vi "plot_data_update.vi"(0 "plotData":i32[][](array[numeric]), 1 "idx start":i32, 2 "length":i32, 3 "AcqData":sgl[](array[numeric]) format="%.2f", 5 "error in (no error)":errorcluster, 6 "max value":sgl format="%.2f", 7 "error rangeViolation":bool=TRUE, 8 "min value":sgl format="%.2f", 9 "error if all equal (false)":bool, 10 "autoScale Y":bool) -> (11 "pixels Y":i32, 13 "pixels X":i32, 14 "plotData out":i32[][](array[numeric]), 15 "updated":bool, 16 "length copy":u32, 17 "dataVal max":sgl format="%.2f", 18 "dataVal min":sgl format="%.2f", 19 "error out":errorcluster)   [LabVIEW 2010, in "OSA.lvclass"]
doc: "Reads the contents of a <B>Thorlabs_OSA_32</B> object.\n\n[GOOP 1.0]"
uses:
  OSA.lvclass
  OSA20X_misc.lvlib
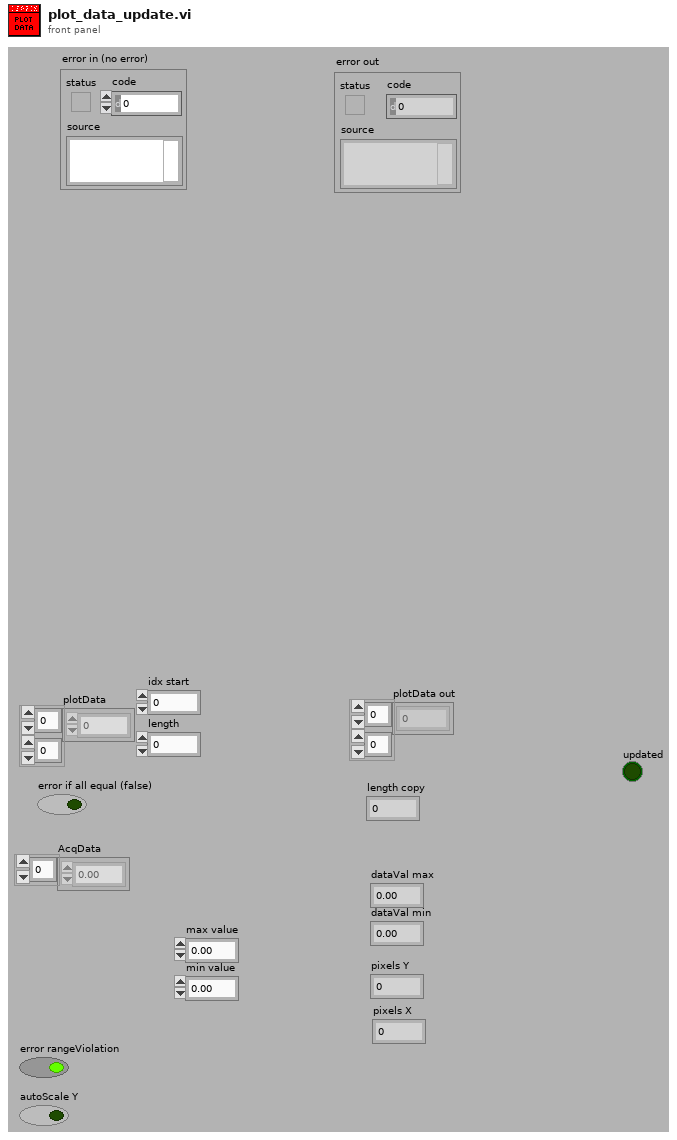
[diagram p1: front panel]
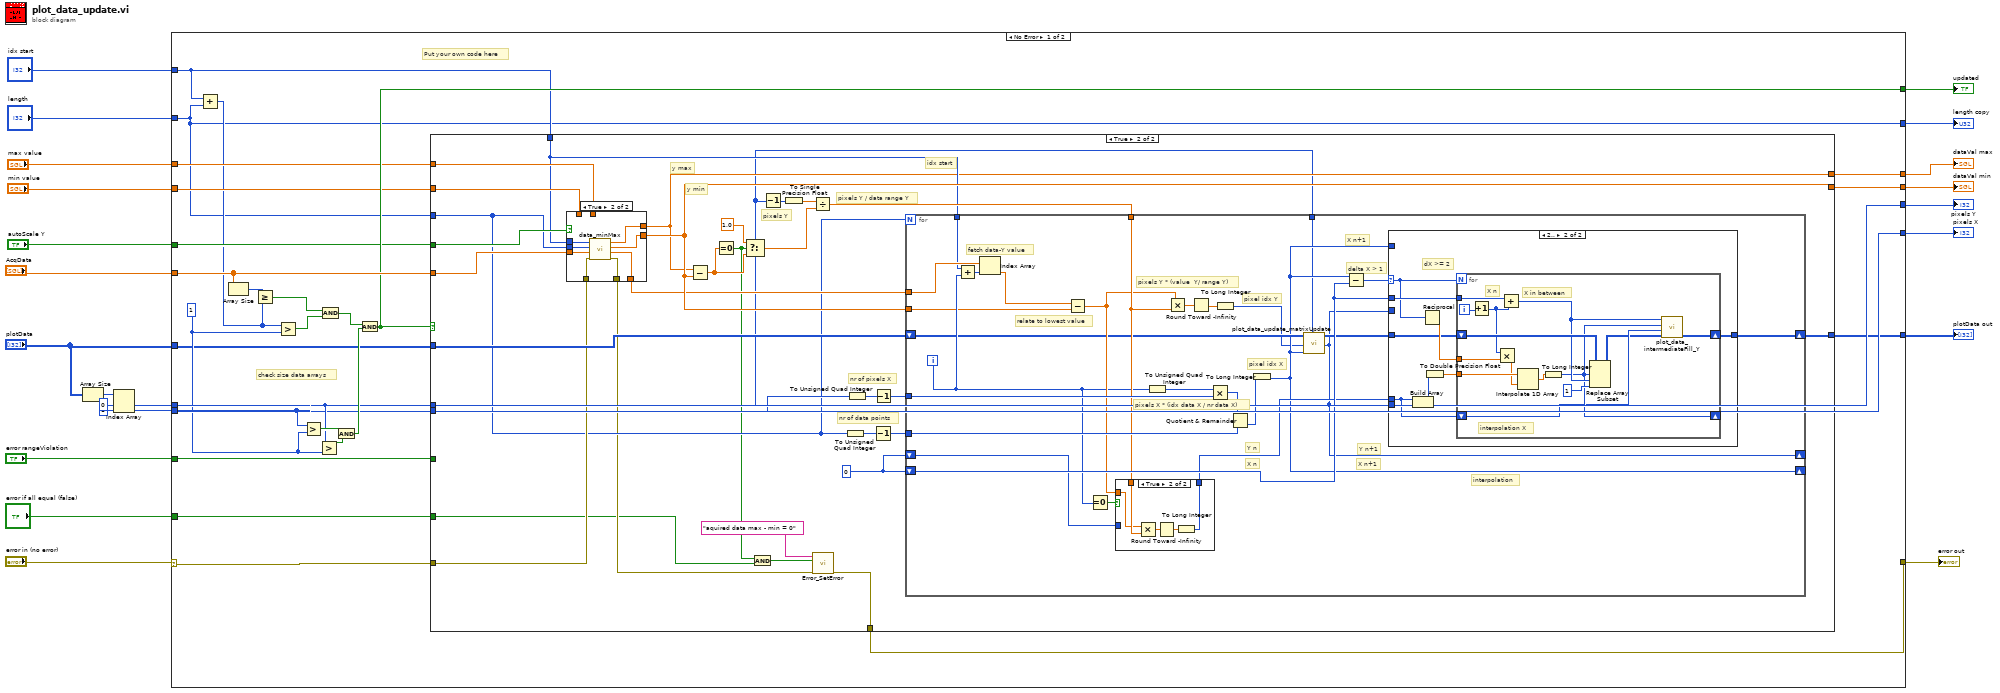
[diagram p0: block diagram]
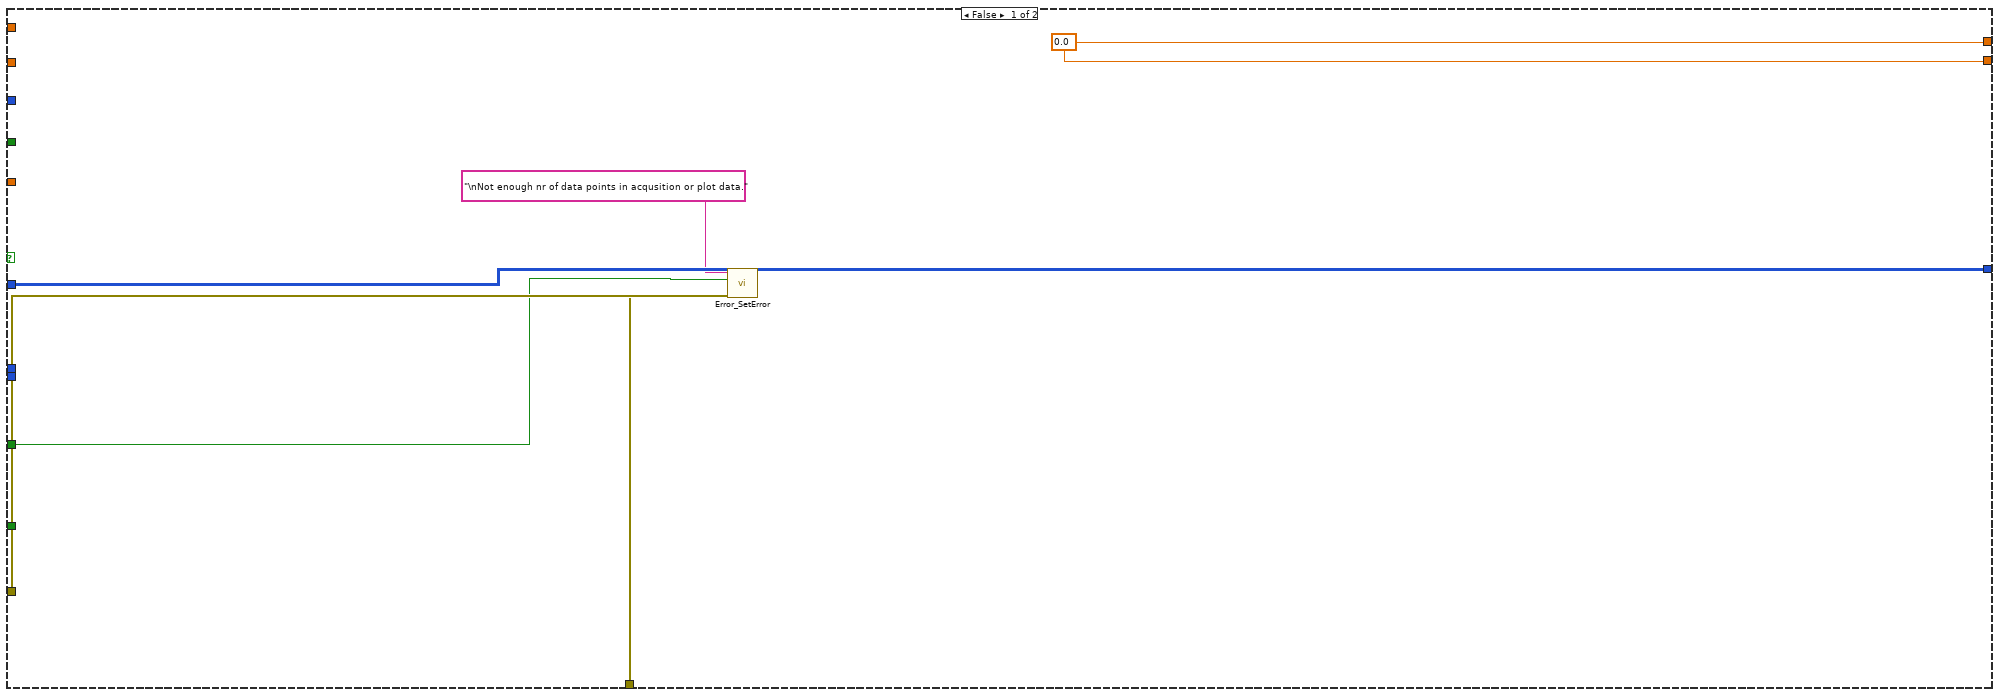
[diagram p2: hidden frame]
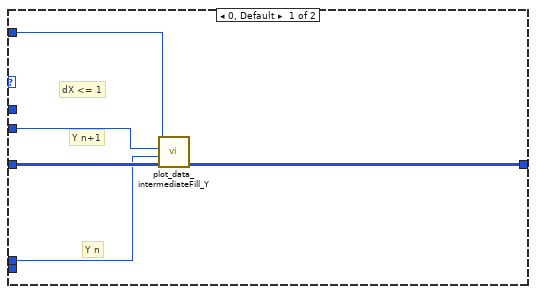
[diagram p5: hidden frame]
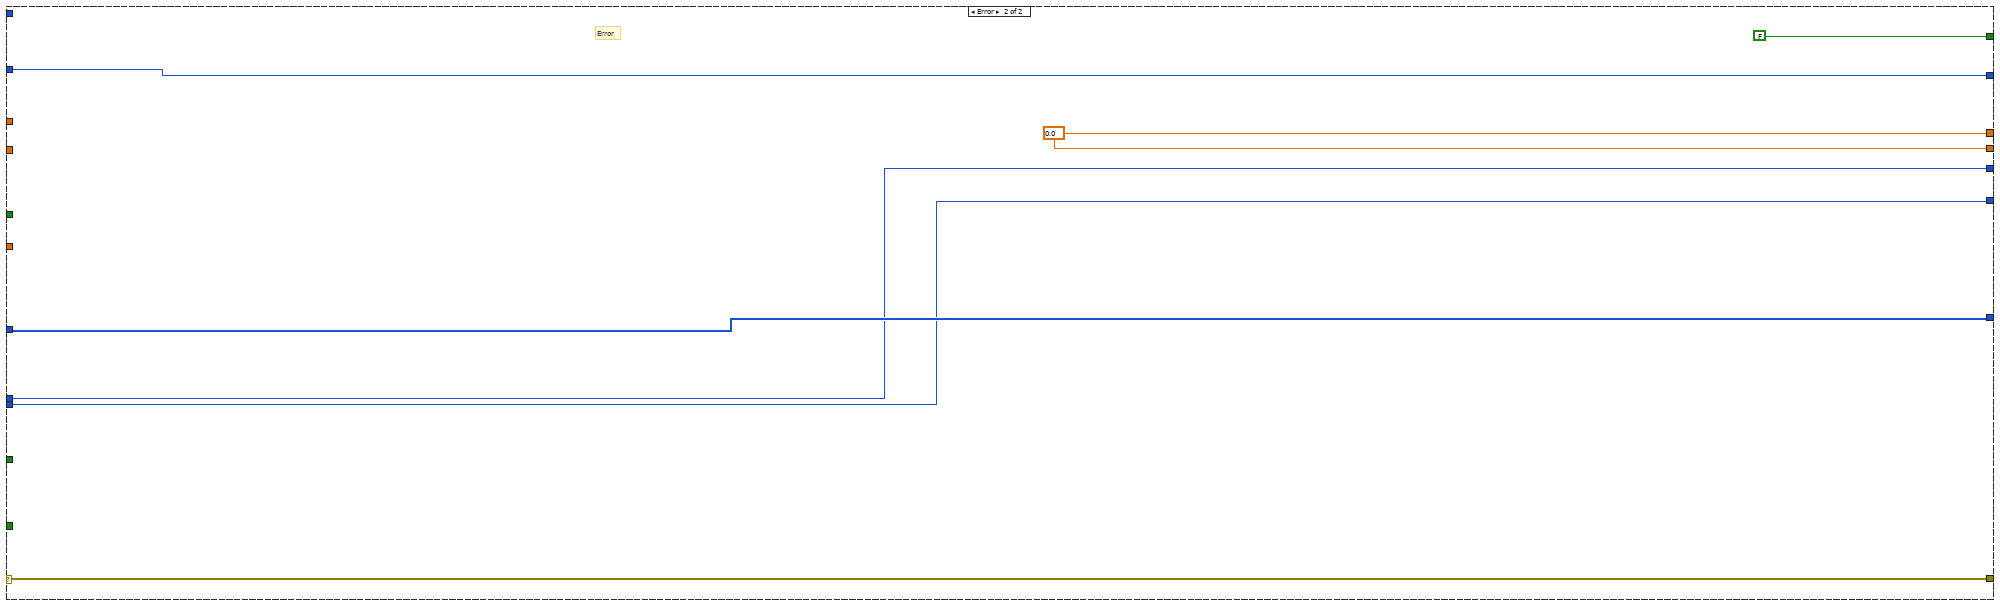
[diagram p6: hidden frame]
diagram:
  n1 = Array Size(array="plotData") -> (size(s)=w15:i32[])
  n2 = Index Array(array=w15, index #1=0 ("index"), index #2=1 ("index")) -> (element #1=w12:i32, element #2=w11:i32)
  n3 = case shown="No Error" "error in (no error)" {
    selector: "error in (no error)" -> [w40 w166]
    tunnel: [w39 w166] -> w23
    tunnel: "AcqData" -> [w49 _]
    tunnel: "plotData" -> [w34 w165]
    tunnel: [w33 w165] -> w2
    tunnel: [w38 w164] -> w20
    tunnel: [w37 w164] -> w19
    tunnel: [w25 w160] -> w18
    tunnel: [w36 w163] -> w17
    tunnel: [w35 w162] -> w16
    tunnel: w12 -> [w36 w163]
    tunnel: w11 -> [w35 w162]
    tunnel: "error rangeViolation" -> [w32 _]
    tunnel: [w31 FALSE] -> w8
    tunnel: "min value" -> [w30 _]
    tunnel: "max value" -> [w29 _]
    tunnel: "autoScale Y" -> [w28 _]
    tunnel: "idx start" -> [w27 _]
    tunnel: "length" -> [w25 w160]
    tunnel: "error if all equal (false)" -> [w24 _]
    frame No Error {
      w45 = u32 1 ("y")
      # "check size data arrays"
      # "Put your own code here"
      n4 = Add(x=w27, y=w25) -> (x+y=w26:i32)
      n5 = Array Size(array=w49) -> (size(s)=w48:i32)
      n6 = Greater Or Equal?(x=w48, y=w26) -> (x >= y?=w47:bool)
      n7 = Greater?(x=w26, y=w45) -> (0:w46:bool)
      n8 = Greater?(x=w35, y=w45) -> (0:w43:bool)
      n9 = Greater?(x=w36, y=w45) -> (0:w44:bool)
      n10 = And(x=w47, y=w46) -> (x .and. y?=w41:bool)
      n11 = And(x=w43, y=w44) -> (x .and. y?=w42:bool)
      n12 = And(x=w41, y=w42) -> (x .and. y?=w31:bool)
      n13 = case shown="True" w31 {
        tunnel: [w53 w86] -> w33
        tunnel: w34 -> [w53 w85]
        tunnel: w49 -> [_ w78]
        tunnel: w36 -> [_ w65]
        tunnel: w35 -> [_ w84]
        tunnel: w40 -> [w55 w79]
        tunnel: [w54 w60] -> w39
        tunnel: w25 -> [_ w67]
        tunnel: [w51 w66] -> w38
        tunnel: [w51 w80] -> w37
        tunnel: w32 -> [w50 _]
        tunnel: w30 -> [_ w83]
        tunnel: w29 -> [_ w82]
        tunnel: w28 -> [_ w81]
        tunnel: w27 -> [_ w68]
        tunnel: w24 -> [_ w58]
        frame False {
          w51 = sgl 0.0
          n14 = call "Error_SetError.vi"("error in"=w55, "status (true)"=w50, "source(\"\")"="\nNot enough nr of data points in acqusition or plot data." ("source(\"\")")) -> ("error out"=w54:errorcluster)  [unwired: 4 in]
        }
        frame True {
          w70 = 0
          # "y min"
          # "y max"
          # "idx start"
          # "pixels Y / data range Y"
          # "nr of data points"
          # "nr of pixels X"
          # "pixels Y"
          n15 = case shown="True" w81 {
            tunnel: w83 -> [w89 _]
            tunnel: w82 -> [w90 _]
            tunnel: w78 -> [w88 w98]
            tunnel: [w88 w97] -> w69
            tunnel: [w90 w96] -> w66
            tunnel: [w89 w95] -> w80
            tunnel: w79 -> [w87 w94]
            tunnel: [w87 w93] -> w61
            tunnel: w68 -> [_ w92]
            tunnel: w67 -> [_ w91]
            frame False {
            }
            frame True {
              n16 = call "data_minMax.vi"("error in (no error)"=w94, "AcqData"=w98, "length"=w91, "idx start"=w92) -> ("error out"=w93:errorcluster, "dataOut"=w97:sgl[], "min"=w95:sgl, "max"=w96:sgl)  [unwired: 4 in]
            }
          }
          n17 = Subtract(x=w66, y=w80) -> (x-y=w63:sgl)
          n18 = Equal To 0?(x=w63) -> (x = 0?=w57:bool)
          n19 = Select(t=sgl 1.0 ("x-y"), s=w57, f=w63) -> (s? t:f=w62:sgl)
          n20 = And(x=w57, y=w58) -> (x .and. y?=w56:bool)
          n21 = Decrement(x=w65) -> (x-1=w76:i32)
          n22 = To Single Precision Float(number=w76) -> (single precision float=w77:sgl)
          n23 = Divide(x=w77, y=w62) -> (x/y=w71:sgl)
          n24 = call "Error_SetError.vi"("error in"=w61, "status (true)"=w56, "source(\"\")"="aquired data max - min = 0" ("source(\"\")")) -> ("error out"=w60:errorcluster)  [unwired: 4 in]
          n25 = To Unsigned Quad Integer(1:w67) -> (0:w72:u64)
          n26 = To Unsigned Quad Integer(1:w84) -> (0:w73:u64)
          n27 = Decrement(x=w72) -> (x-1=w75:u64)
          n28 = Decrement(x=w73) -> (x-1=w74:u64)
          n29 = for {
            N: w67 -> [_]
            shift-right: [w122] -> w86
            shift-left: w85 -> [w105]
            tunnel: w69 -> [w113]
            tunnel: w74 -> [w125]
            tunnel: w75 -> [w124]
            tunnel: w71 -> [w121]
            shift-right: [w101] -> _
            shift-left: w70 -> [w120]
            shift-right: [w103] -> _
            shift-left: w70 -> [w123]
            tunnel: w80 -> [w108]
            tunnel: w68 -> [w110]
            tunnel: w65 -> [w100]
            i -> [w111]
            # "X n+1"
            # "pixels X * (idx data X / nr data X)"
            # "pixels Y * (value  Y/ range Y)"
            # "relate to lowest value"
            # "fetch data-Y value"
            # "X n"
            # "Y n"
            # "pixel idx X"
            # "pixel idx Y"
            # "delta X > 1"
            # "interpolation"
            # "Y n+1"
            # "X n+1"
            n30 = Add(x=w110, y=w111) -> (x+y=w112:i32)
            n31 = Index Array(array=w113, index=w112) -> (element=w109:sgl)
            n32 = Subtract(x=w109, y=w108) -> (x-y=w114:sgl)
            n33 = Equal To 0?(x=w111) -> (x = 0?=w116:bool)
            n34 = case shown="True" w116 {
              tunnel: w121 -> [_ w129]
              tunnel: w114 -> [_ w128]
              tunnel: [w126 w127] -> w115
              tunnel: w120 -> [w126 _]
              frame False {
              }
              frame True {
                n35 = Multiply(x=w128, y=w129) -> (x*y=w130:sgl)
                n36 = Round Toward -Infinity(1:w130) -> (0:w131:sgl)
                n37 = To Long Integer(number=w131) -> (32bit integer=w127:i32)
              }
            }
            n38 = To Unsigned Quad Integer(1:w111) -> (0:w99:u64)
            n39 = Multiply(x=w114, y=w121) -> (x*y=w107:sgl)
            n40 = Round Toward -Infinity(1:w107) -> (0:w106:sgl)
            n41 = Multiply(x=w99, y=w125) -> (x*y=w119:u64)
            n42 = To Long Integer(number=w106) -> (32bit integer=w102:i32)
            n43 = Quotient & Remainder(x=w119, y=w124) -> (floor(x/y)=w118:u64)  [unwired: 1 out]
            n44 = To Long Integer(number=w118) -> (32bit integer=w103:i32)
            n45 = call "plot_data_update_matrixUpdate.vi"("XY plot"=w105, "idx Y"=w102, "idx X"=w103, "Y size"=w100) -> ("XY plot out"=w104:i32[][], "idx Y out"=w101:i32)  [unwired: 13 in, 1 out]
            n46 = Subtract(x=w103, y=w123) -> (x-y=w117:i32)
            n47 = case shown="2.." w117 {
              selector: w117 -> [_ w137]
              tunnel: w115 -> [w133 w139]
              tunnel: w101 -> [_ w145]
              tunnel: [w132 w142] -> w122
              tunnel: w104 -> [w135 w140]
              tunnel: w101 -> [w134 _]
              tunnel: w103 -> [w136 _]
              tunnel: w123 -> [_ w138]
              frame 0, Default {
                # "Y n"
                # "Y n+1"
                # "dX <= 1"
                n48 = call "plot_data_intermediateFill_Y.vi"("plotData"=w135, "idx Y (n)"=w133, "idx Y (n+1)"=w134, "idx X"=w136) -> ("plotData out"=w132:i32[][])  [unwired: 7 in]
              }
              frame 2.. {
                # "dX >= 2"
                n49 = Build Array(w139, w145) -> (w144:i32[])
                n50 = Reciprocal(x=w137) -> (1/x=w143:dbl)
                n51 = To Double Precision Float(number=w144) -> (double precision float=w141:dbl[])
                n52 = for {
                  N: w137 -> [_]
                  shift-right: [w147] -> w142
                  shift-left: w140 -> [w158]
                  tunnel: w138 -> [w159]
                  tunnel: w141 -> [w157]
                  tunnel: w143 -> [w154]
                  shift-right: [w150] -> _
                  shift-left: w139 -> [w149]
                  i -> [w156]
                  # "X n"
                  # "X in between"
                  # "interpolation X"
                  n53 = Increment(x=w156) -> (x+1=w155:i32)
                  n54 = Multiply(x=w155, y=w154) -> (x*y=w153:dbl)
                  n55 = Add(x=w159, y=w155) -> (x+y=w151:i32)
                  n56 = Interpolate 1D Array(1:w153, 2:w157) -> (0:w146:dbl)
                  n57 = To Long Integer(number=w146) -> (32bit integer=w150:i32)
                  n58 = Replace Array Subset(array=w158, new element=1 ("new element/subarray"), index (row)=w150, index (col)=w151) -> (w148:i32[][])
                  n59 = call "plot_data_intermediateFill_Y.vi"("plotData"=w148, "idx Y (n)"=w149, "idx Y (n+1)"=w150, "idx X"=w151) -> ("plotData out"=w147:i32[][])  [unwired: 7 in]
                }
              }
            }
          }
        }
      }
    }
    frame Error {
      w164 = sgl 0.0
      # "Error"
    }
  }
  "error out" <- w23
  "plotData out" <- w2
  "dataVal max" <- w20
  "dataVal min" <- w19
  "length copy" <- w18
  "pixels Y" <- w17
  "pixels X" <- w16
  "updated" <- w8
